vi "fpga.sandbox.vi"() -> ()   [LabVIEW 2022 SP3]
uses:
  bats.parser/data.ctl
  <vilib>/Platform/TimedLoop/XDataNode/timing_clust.ctl
  <vilib>/Platform/TimedLoop/XDataNode/nitl_modes.ctl
  <vilib>/Platform/TimedLoop/XDataNode/wakeup.ctl
  <vilib>/rvi/Emulation/niFpgaSctlEmulationGetInTimedLoop.vi
  <vilib>/rvi/Emulation/niFpgaEmulationReportErrorSimple.vi
  <vilib>/rvi/Emulation/niFpgaGetClockAttributes.vi
  <vilib>/rvi/Emulation/niFpgaCriticalErrorInLSC.vi
  <vilib>/rvi/interface/RandomDataEmulation/nirviRandomDataMultiElementFPGAFIFO.vi
  <instcachedir>/0/nirviRandomDataMultiElementFPGAFIFO_3E9965BA1FAD4E7B8DABA31768A09B1F.lvgen/nirviRandomDataMultiElementFPGAFIFO_3E9965BA1FAD4E7B8DABA31768A09B1F_003.vi
  <vilib>/rvi/interface/RandomDataEmulation/niFpgaRandomDataHandleErrors.vi
  <vilib>/Platform/TimedLoop/XDataNode/XDataNode.xnode
  <vilib>/rvi/DataTransferAndStorage/Container/XNode/niFpgaContainer.xnode
  <vilib>/rvi/interface/RandomDataEmulation/nirviRandomDataFpgaMultiElementTemplate.vi
  <vilib>/Platform/TimedLoop/XDataNode/XDNodeRunTimeDep.lvlib
panel:
  out "Count":i16
  out "data":T1 {"byte" format="%.0x"}
  out "number":u8 format="%.0x"
  in  "Ready for Output":bool
  out "Element":u16[](array[numeric]) format="%.0x"
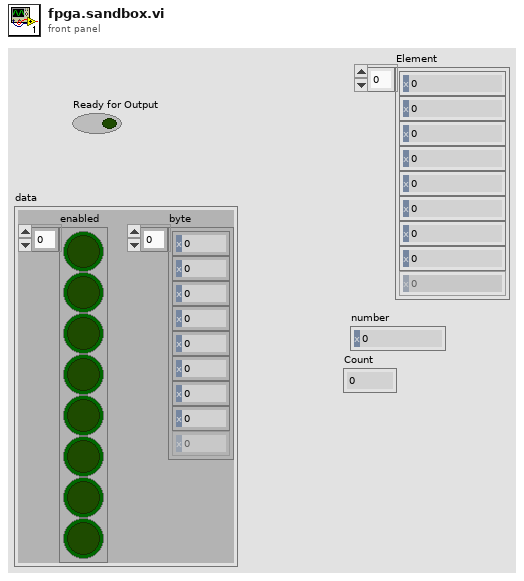
[diagram p1: front panel]
types:
  T1 = typedef "data.ctl" = cluster{"enabled":bool[], "byte":u8[]}
  T2 = typedef "XDNodeRunTimeDep.lvlib/timing_clust.ctl" = cluster{"Expected End [f-1]":u64, "Actual End [f-1]":u64, "Finished Late? [f-1]":bool, "Expected End [i-1]":u64, "Actual End [i-1]":u64, "Finished Late? [i-1]":bool, "Expected Start [i]":u64, "Actual Start [i]":u64, "Expected Start [f]":u64, "Actual Start [f]":u64, "Source Name":string, "Structure Name":string, "Period":i64, "Deadline":i64, "Offset":i64, "Start":i64, "Priority":i32, "Timeout":i32, "Mode":T3, "Wakeup Reason":T4, "Error":errorcluster, "Source Type":string, "Secondary Source Type":string, "Global End Time":u64, "Global Start Time":u64, "Frame Duration":u64, "Iteration Duration":u64, "Assigned CPU":i32, "I/O Scan Engine Mode":u32}
  T3 = typedef "XDNodeRunTimeDep.lvlib/nitl_modes.ctl" = enum32{"No Change", "Process missed periods, maintain original phase", "Discard missed periods, maintain original phase", "Process missed periods, ignore original phase", "Discard missed periods, ignore original phase"}
  T4 = typedef "XDNodeRunTimeDep.lvlib/wakeup.ctl" = enum32{"Normal", "Aborted", "Asynchronous wakeup", "Timing source error", "Timed loop error", "Timeout"}
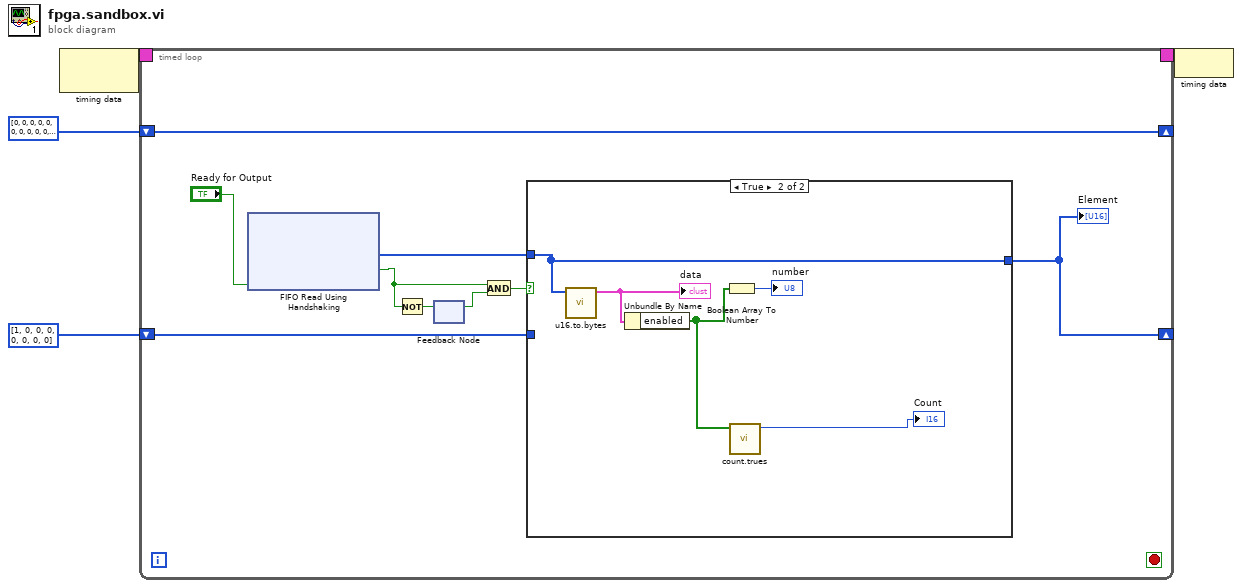
[diagram p0: block diagram]
diagram:
  n1 = node-c288() -> (w4:T2)  [unwired: 1 in]
  n2 = timed-loop {
    timing: w4 -> [_]
    timing-out: [_] -> w3
    shift-right: [w13] -> _
    shift-left: u8[] [0, 0, 0, 0, 0, 0, 0, 0, 0, 0, 0, 0, 0, 0, 0, 0] -> [w13]
    shift-right: [w5] -> _
    shift-left: u16[] [1, 0, 0, 0, 0, 0, 0, 0] ("s? t:f") -> [w10]
    stop <- _ stop-if-true
    n3 = xnode "FIFO Read Using Handshaking"("Ready for Output"="Ready for Output") -> ("Element"=w11:u16[], "Output Valid"=w7:bool)  [unwired: 1 in, 1 out]
    n4 = Not(x=w7) -> (.not. x?=w8:bool)
    n5 = feedback-in #1(w8) -> ()
    n6 = feedback #1() -> (w12:bool)  [unwired: 1 in]
    n7 = And(x=w7, y=w12) -> (x .and. y?=w9:bool)
    n8 = case shown="True" w9 {
      tunnel: w11 -> [_ w19]
      tunnel: w10 -> [w14 _]
      tunnel: [w14 w19] -> w5
      frame False {
      }
      frame True {
        n9 = call "u16.to.bytes.vi"("data.u16.in"=w19) -> ("data"=w18:T1)  [unwired: 10 in]
        "data" <- w18
        n10 = Unbundle By Name(w18) -> ("enabled"=w16:bool[])
        n11 = Boolean Array To Number(Boolean array=w16) -> (number=→"number":u8)
        n12 = call "count.trues.vi"("enabled"=w16) -> ("Numeric"=→"Count":u8)  [unwired: 10 in]
      }
    }
    "Element" <- w5
  }
  n13 = node-c288(w3) -> ()
